vi "Read Data.vi"(8 "error in (no error)":errorcluster, 9 "DataType":T1=enum."U8", 10 "Address":string, 11 "Simulated_PLC in":refnum<class "Simulated_PLC.lvclass">) -> (0 "error out":errorcluster, 2 "Data":variant, 3 "Simulated_PLC out":refnum<class "Simulated_PLC.lvclass">)   [LabVIEW 2025, in "Simulated_PLC.lvclass"]
uses:
  Simulated_PLC.lvclass
  PLC_Module/PLC_Module/PLC_Data_Type.ctl
  PLC_Abstr/PLC_Abstr/PLC_Abstr.lvclass
  Simulated_PLC.lvclass/Simulated_PLC.ctl
  PLC_Module/PLC_Module/PLC_Module.lvclass
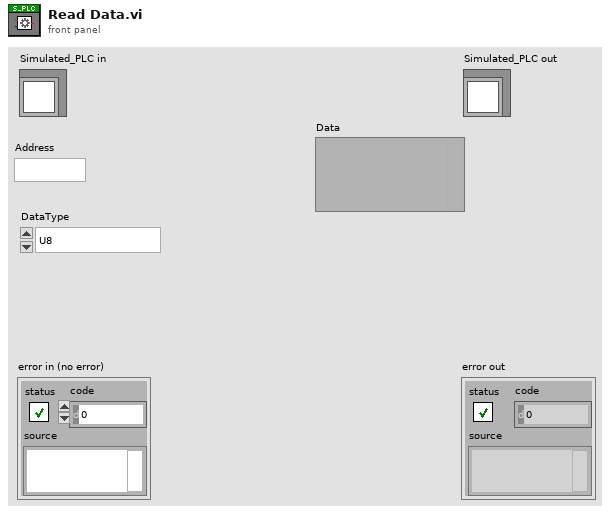
[diagram p1: front panel]
types:
  T1 = typedef "PLC_Module.lvlib/PLC_Module.lvclass/PLC_Data_Type.ctl" = enum16{"Boolean", "Single Float", "U8", "U32", "U32_Array", "String"}
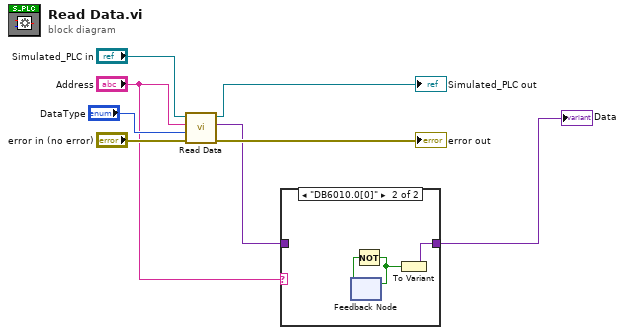
[diagram p0: block diagram]
diagram:
  n1 = call-parent "Read Data.vi"("error in (no error)"="error in (no error)", "DataType"="DataType", "Address"="Address", "PLC_Abstr in"="Simulated_PLC in") -> ("error out"=→"error out":errorcluster, "Data"=w2:variant, "PLC_Abstr out"=→"Simulated_PLC out":refnum<class "Simulated_PLC.lvclass">)  [unwired: 5 in]
  n2 = case shown="\"DB6010.0[0]\"" "Address" {
    tunnel: w2 -> [w9 _]
    tunnel: [w9 w10] -> w1
    frame Default {
    }
    frame "DB6010.0[0]" {
      n3 = feedback #1() -> (w12:bool)  [unwired: 1 in]
      n4 = Not(x=w12) -> (.not. x?=w11:bool)
      n5 = feedback-in #1(w11) -> ()
      n6 = To Variant(anything=w11) -> (Variant=w10:variant)
    }
  }
  "Data" <- w1
